vi "GetSimulatedCameras.vi"(8 "error in (no error)":errorcluster) -> (0 "error out":errorcluster, 3 "Camera Info":T1(array[cluster]))   [LabVIEW 2017, in "IrManageCameras.lvlib"]
uses:
  <vilib>/addons/InsightCM/Devices/Shared/Ir/IrManageCameras/IrManageCameras.lvlib
  <vilib>/addons/InsightCM/Devices/Shared/Ir/IrManageCameras/subVIs/SimConfigRefGlobal.vi
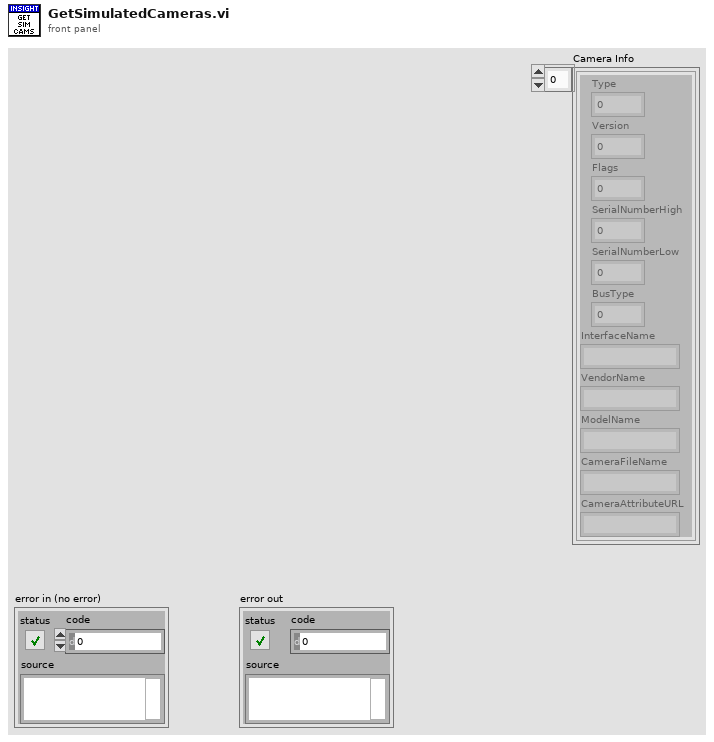
[diagram p1: front panel]
types:
  T1 = cluster{"Type":u32, "Version":u32, "Flags":u32, "SerialNumberHigh":u32, "SerialNumberLow":u32, "BusType":u32, "InterfaceName":string, "VendorName":string, "ModelName":string, "CameraFileName":string, "CameraAttributeURL":string}[]
  T2 = cluster{"Serial Number":string, "Camera Type":string}[]
  T3 = cluster{"Type":u32, "Version":u32, "Flags":u32, "SerialNumberHigh":u32, "SerialNumberLow":u32, "BusType":u32, "InterfaceName":string, "VendorName":string, "ModelName":string, "CameraFileName":string, "CameraAttributeURL":string}
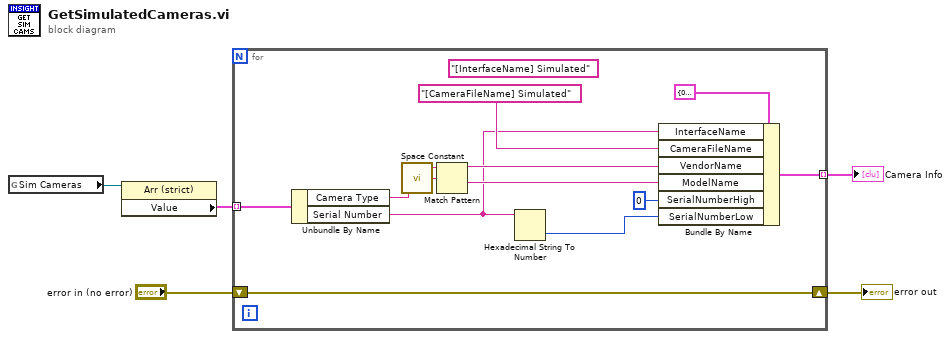
[diagram p0: block diagram]
diagram:
  n1 = global read "SimConfigRefGlobal.vi" "Sim Cameras"() -> (w5:refnum<vi>)
  n2 = property class="Arr (strict)"(reference=w5) -> ("Value"=w4:T2)  [unwired: 1 in, 2 out]
  n3 = for {
    tunnel: w4 -> [w11] mode=indexing
    tunnel: [w9] -> w1 mode=indexing
    shift-right: [w8] -> w2
    shift-left: "error in (no error)" -> [w8]
    (unwired) "[InterfaceName] Simulated" ("InterfaceName")
    n4 = Unbundle By Name(w11) -> ("Camera Type"=w17:string, "Serial Number"=w6:string)
    n5 = call <vilib>:"Space Constant.vi"() -> ("String"=w16:string)
    n6 = Match Pattern(string=w17, regular expression=w16) -> (before substring=w15:string, after substring=w14:string)  [unwired: 1 in, 2 out]
    n7 = Hexadecimal String To Number(string=w6) -> (number=w12:u32)  [unwired: 2 in, 1 out]
    n8 = Bundle By Name(cluster=T3 {"Type"=0, "Version"=0, "Flags"=0, "SerialNumberHigh"=0, "SerialNumberLow"=0, "BusType"=0, "InterfaceName"="", "VendorName"="", "ModelName"="", "CameraFileName"="", "CameraAttributeURL"=""} ("Camera"), "InterfaceName"=w6, "CameraFileName"="[CameraFileName] Simulated" ("InterfaceName"), "VendorName"=w15, "ModelName"=w14, "SerialNumberHigh"=u32 0, "SerialNumberLow"=w12) -> (w9:T3)
  }
  "error out" <- w2
  "Camera Info" <- w1
